vi "Autonomous Independent.vi"   [LabVIEW 2020]
doc: "This VI is called when autonomous begins, and will automatically be terminated when autonomous ends. You can carry out timed or sensor driven robot movement independently without needing to return to the caller."
uses:
  <vilib>/Rock Robotics/Network Tables/NT Read String.vi
  Robot Global Data.vi
panel:
  # "Be sure to right-click and choose Data Operations>>Make Current Value default if you want to save the array values with the VI"
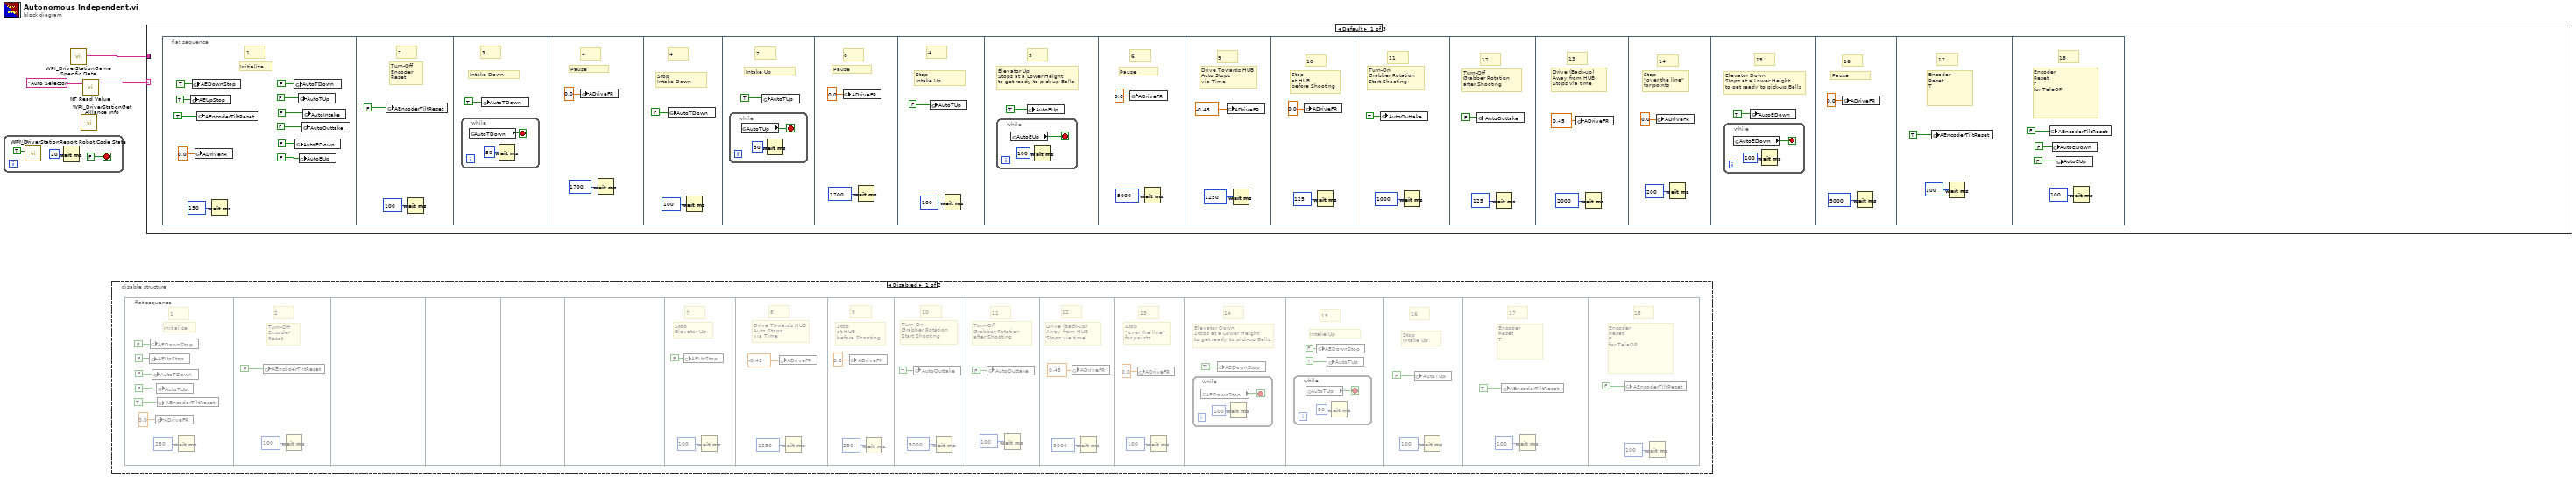
[diagram p0: block diagram]
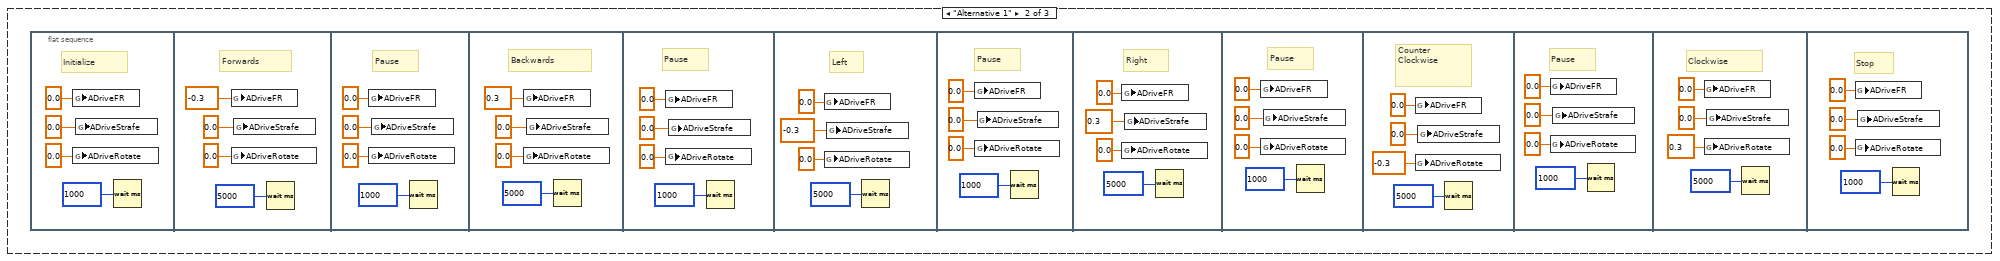
[diagram p3: hidden frame]
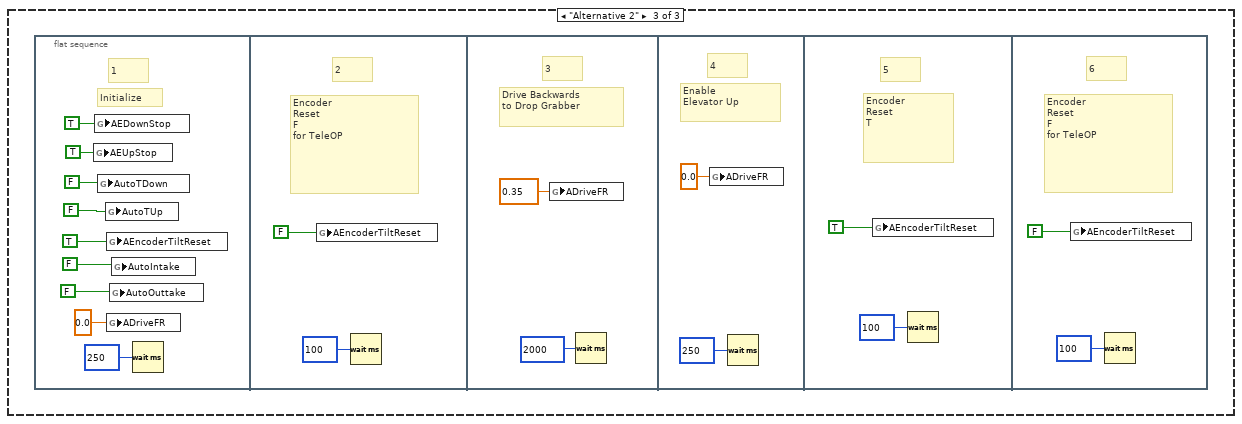
[diagram p4: hidden frame]
diagram:
  n1 = while {
    stop <- FALSE stop-if-true
    n2 = call <vilib>:"WPI_DriverStationReport Robot Code State.vi"("Autonomous"=TRUE) -> ()  [unwired: 10 in, 1 out]
    n3 = Wait (ms)(milliseconds to wait=u32 20) -> ()  [unwired: 1 out]
  }
  n4 = call <vilib>:"WPI_DriverStationGame Specific Data.vi"() -> ("Game Specific Data"=w1:string)  [unwired: 11 in]
  n5 = call <vilib>:"WPI_DriverStationGet Alliance Info.vi"() -> ()  [unwired: 12 out]
  n6 = call-poly <vilib>:"NT Read Value.vi"("Name"="Auto Selector") -> ("String"=w2:string)  [unwired: 9 in, 1 out]
  n7 = disable-structure shown="Disabled" {
    frame Disabled {
      n8 = flat-sequence {
        frame #0 {
          # "1"
          # "Initialize"
          n9 = global write "Robot Global Data.vi" "AEUpStop"(FALSE) -> ()
          n10 = global write "Robot Global Data.vi" "AEDownStop"(FALSE) -> ()
          n11 = global write "Robot Global Data.vi" "AutoTDown"(FALSE) -> ()
          n12 = global write "Robot Global Data.vi" "ADriveFR"(0.0 ("ADriveFR")) -> ()
          n13 = global write "Robot Global Data.vi" "AutoTUp"(FALSE) -> ()
          n14 = global write "Robot Global Data.vi" "AEncoderTiltReset"(TRUE) -> ()
          n15 = Wait (ms)(milliseconds to wait=u32 250) -> ()  [unwired: 1 out]
        }
        frame #1 {
          # "2"
          # "Turn-Off\nEncoder\nReset"
          n16 = global write "Robot Global Data.vi" "AEncoderTiltReset"(FALSE) -> ()
          n17 = Wait (ms)(milliseconds to wait=u32 100) -> ()  [unwired: 1 out]
        }
        frame #2 {
        }
        frame #3 {
        }
        frame #4 {
        }
        frame #5 {
        }
        frame #6 {
          # "7"
          # "Stop\nElevator Up"
          n18 = global write "Robot Global Data.vi" "AEUpStop"(FALSE) -> ()
          n19 = Wait (ms)(milliseconds to wait=u32 100) -> ()  [unwired: 1 out]
        }
        frame #7 {
          # "8"
          # "Drive Towards HUB\nAuto Stops\nvia Time"
          n20 = global write "Robot Global Data.vi" "ADriveFR"(-0.45 ("ADriveFR")) -> ()
          n21 = Wait (ms)(milliseconds to wait=u32 1250) -> ()  [unwired: 1 out]
        }
        frame #8 {
          # "9"
          # "Stop\nat HUB\nbefore Shooting"
          n22 = global write "Robot Global Data.vi" "ADriveFR"(0.0 ("ADriveFR")) -> ()
          n23 = Wait (ms)(milliseconds to wait=u32 250) -> ()  [unwired: 1 out]
        }
        frame #9 {
          # "10"
          # "Turn-On\nGrabber Rotation\nStart Shooting"
          n24 = global write "Robot Global Data.vi" "AutoOuttake"(TRUE ("AutoOuttake")) -> ()
          n25 = Wait (ms)(milliseconds to wait=u32 3000) -> ()  [unwired: 1 out]
        }
        frame #10 {
          # "11"
          # "Turn-Off\nGrabber Rotation\nafter Shooting"
          n26 = global write "Robot Global Data.vi" "AutoOuttake"(FALSE ("AutoOuttake")) -> ()
          n27 = Wait (ms)(milliseconds to wait=u32 100) -> ()  [unwired: 1 out]
        }
        frame #11 {
          # "12"
          # "Drive (Back-up)\nAway from HUB\nStops via time"
          n28 = global write "Robot Global Data.vi" "ADriveFR"(0.45 ("ADriveFR")) -> ()
          n29 = Wait (ms)(milliseconds to wait=u32 3000) -> ()  [unwired: 1 out]
        }
        frame #12 {
          # "13"
          # "Stop\n\"over the line\"\nfor points"
          n30 = global write "Robot Global Data.vi" "ADriveFR"(0.0 ("ADriveFR")) -> ()
          n31 = Wait (ms)(milliseconds to wait=u32 100) -> ()  [unwired: 1 out]
        }
        frame #13 {
          # "14"
          # "Elevator Down\nStops at a Lower Height\nto get ready to pick-up Balls"
          n32 = while {
            stop <- w31 stop-if-true
            n33 = global read "Robot Global Data.vi" "AEDownStop"() -> (w31:bool)
            n34 = Wait (ms)(milliseconds to wait=u32 100) -> ()  [unwired: 1 out]
          }
          n35 = global write "Robot Global Data.vi" "AEDownStop"(TRUE) -> ()
        }
        frame #14 {
          # "Intake Up"
          # "15"
          n36 = while {
            stop <- w35 stop-if-true
            n37 = global read "Robot Global Data.vi" "AutoTUp"() -> (w35:bool)
            n38 = Wait (ms)(milliseconds to wait=u32 50) -> ()  [unwired: 1 out]
          }
          n39 = global write "Robot Global Data.vi" "AEDownStop"(FALSE) -> ()
          n40 = global write "Robot Global Data.vi" "AutoTUp"(TRUE) -> ()
        }
        frame #15 {
          # "Stop\nIntake Up"
          # "16"
          n41 = global write "Robot Global Data.vi" "AutoTUp"(FALSE) -> ()
          n42 = Wait (ms)(milliseconds to wait=u32 100) -> ()  [unwired: 1 out]
        }
        frame #16 {
          # "17"
          # "Encoder\nReset\nT"
          n43 = global write "Robot Global Data.vi" "AEncoderTiltReset"(TRUE) -> ()
          n44 = Wait (ms)(milliseconds to wait=u32 100) -> ()  [unwired: 1 out]
        }
        frame #17 {
          # "18"
          # "Encoder\nReset\nF \nfor TeleOP"
          n45 = global write "Robot Global Data.vi" "AEncoderTiltReset"(FALSE) -> ()
          n46 = Wait (ms)(milliseconds to wait=u32 100) -> ()  [unwired: 1 out]
        }
      }
    }
    frame Enabled {
    }
  }
  n47 = case shown="Default" w2 {
    tunnel: w1 -> [_ _ _]
    frame Default {
      n48 = flat-sequence {
        frame #0 {
          # "1"
          # "Initialize"
          n49 = global write "Robot Global Data.vi" "AEUpStop"(TRUE) -> ()
          n50 = global write "Robot Global Data.vi" "AEDownStop"(TRUE) -> ()
          n51 = global write "Robot Global Data.vi" "ADriveFR"(0.0 ("ADriveFR")) -> ()
          n52 = global write "Robot Global Data.vi" "AEncoderTiltReset"(TRUE) -> ()
          n53 = Wait (ms)(milliseconds to wait=u32 150) -> ()  [unwired: 1 out]
          n54 = global write "Robot Global Data.vi" "AutoTDown"(FALSE) -> ()
          n55 = global write "Robot Global Data.vi" "AutoEDown"(FALSE) -> ()
          n56 = global write "Robot Global Data.vi" "AutoTUp"(FALSE) -> ()
          n57 = global write "Robot Global Data.vi" "AutoEUp"(FALSE) -> ()
          n58 = global write "Robot Global Data.vi" "AutoOuttake"(FALSE) -> ()
          n59 = global write "Robot Global Data.vi" "AutoIntake"(FALSE) -> ()
        }
        frame #1 {
          # "2"
          # "Turn-Off\nEncoder\nReset"
          n60 = global write "Robot Global Data.vi" "AEncoderTiltReset"(FALSE) -> ()
          n61 = Wait (ms)(milliseconds to wait=u32 100) -> ()  [unwired: 1 out]
        }
        frame #2 {
          # "Intake Down"
          # "3"
          n62 = while {
            stop <- w57 stop-if-true
            n63 = global read "Robot Global Data.vi" "AutoTDown"() -> (w57:bool)
            n64 = Wait (ms)(milliseconds to wait=u32 50) -> ()  [unwired: 1 out]
          }
          n65 = global write "Robot Global Data.vi" "AutoTDown"(TRUE) -> ()
        }
        frame #3 {
          # "4"
          # "Pause"
          n66 = global write "Robot Global Data.vi" "ADriveFR"(0.0 ("ADriveFR")) -> ()
          n67 = Wait (ms)(milliseconds to wait=u32 1700) -> ()  [unwired: 1 out]
        }
        frame #4 {
          # "Stop \nIntake Down"
          # "4"
          n68 = global write "Robot Global Data.vi" "AutoTDown"(FALSE) -> ()
          n69 = Wait (ms)(milliseconds to wait=u32 100) -> ()  [unwired: 1 out]
        }
        frame #5 {
          # "Intake Up"
          # "7"
          n70 = while {
            stop <- w64 stop-if-true
            n71 = global read "Robot Global Data.vi" "AutoTUp"() -> (w64:bool)
            n72 = Wait (ms)(milliseconds to wait=u32 50) -> ()  [unwired: 1 out]
          }
          n73 = global write "Robot Global Data.vi" "AutoTUp"(TRUE) -> ()
        }
        frame #6 {
          # "8"
          # "Pause"
          n74 = global write "Robot Global Data.vi" "ADriveFR"(0.0 ("ADriveFR")) -> ()
          n75 = Wait (ms)(milliseconds to wait=u32 1700) -> ()  [unwired: 1 out]
        }
        frame #7 {
          # "Stop \nIntake Up"
          # "4"
          n76 = global write "Robot Global Data.vi" "AutoTUp"(FALSE) -> ()
          n77 = Wait (ms)(milliseconds to wait=u32 100) -> ()  [unwired: 1 out]
        }
        frame #8 {
          # "5"
          # "Elevator Up\nStops at a Lower Height\nto get ready to pick-up Balls"
          n78 = while {
            stop <- w71 stop-if-true
            n79 = global read "Robot Global Data.vi" "AutoEUp"() -> (w71:bool)
            n80 = Wait (ms)(milliseconds to wait=u32 100) -> ()  [unwired: 1 out]
          }
          n81 = global write "Robot Global Data.vi" "AutoEUp"(TRUE) -> ()
        }
        frame #9 {
          # "6"
          # "Pause"
          n82 = global write "Robot Global Data.vi" "ADriveFR"(0.0 ("ADriveFR")) -> ()
          n83 = Wait (ms)(milliseconds to wait=u32 5000) -> ()  [unwired: 1 out]
        }
        frame #10 {
          # "9"
          # "Drive Towards HUB\nAuto Stops\nvia Time"
          n84 = global write "Robot Global Data.vi" "ADriveFR"(-0.45 ("ADriveFR")) -> ()
          n85 = Wait (ms)(milliseconds to wait=u32 1250) -> ()  [unwired: 1 out]
        }
        frame #11 {
          # "10"
          # "Stop\nat HUB\nbefore Shooting"
          n86 = global write "Robot Global Data.vi" "ADriveFR"(0.0 ("ADriveFR")) -> ()
          n87 = Wait (ms)(milliseconds to wait=u32 125) -> ()  [unwired: 1 out]
        }
        frame #12 {
          # "11"
          # "Turn-On\nGrabber Rotation\nStart Shooting"
          n88 = global write "Robot Global Data.vi" "AutoOuttake"(TRUE ("AutoOuttake")) -> ()
          n89 = Wait (ms)(milliseconds to wait=u32 1000) -> ()  [unwired: 1 out]
        }
        frame #13 {
          # "12"
          # "Turn-Off\nGrabber Rotation\nafter Shooting"
          n90 = global write "Robot Global Data.vi" "AutoOuttake"(FALSE ("AutoOuttake")) -> ()
          n91 = Wait (ms)(milliseconds to wait=u32 125) -> ()  [unwired: 1 out]
        }
        frame #14 {
          # "13"
          # "Drive (Back-up)\nAway from HUB\nStops via time"
          n92 = global write "Robot Global Data.vi" "ADriveFR"(0.45 ("ADriveFR")) -> ()
          n93 = Wait (ms)(milliseconds to wait=u32 2000) -> ()  [unwired: 1 out]
        }
        frame #15 {
          # "14"
          # "Stop\n\"over the line\"\nfor points"
          n94 = global write "Robot Global Data.vi" "ADriveFR"(0.0 ("ADriveFR")) -> ()
          n95 = Wait (ms)(milliseconds to wait=u32 200) -> ()  [unwired: 1 out]
        }
        frame #16 {
          # "15"
          # "Elevator Down\nStops at a Lower Height\nto get ready to pick-up Balls"
          n96 = while {
            stop <- w88 stop-if-true
            n97 = global read "Robot Global Data.vi" "AutoEDown"() -> (w88:bool)
            n98 = Wait (ms)(milliseconds to wait=u32 100) -> ()  [unwired: 1 out]
          }
          n99 = global write "Robot Global Data.vi" "AutoEDown"(TRUE) -> ()
        }
        frame #17 {
          # "16"
          # "Pause"
          n100 = global write "Robot Global Data.vi" "ADriveFR"(0.0 ("ADriveFR")) -> ()
          n101 = Wait (ms)(milliseconds to wait=u32 5000) -> ()  [unwired: 1 out]
        }
        frame #18 {
          # "17"
          # "Encoder\nReset\nT"
          n102 = global write "Robot Global Data.vi" "AEncoderTiltReset"(TRUE) -> ()
          n103 = Wait (ms)(milliseconds to wait=u32 100) -> ()  [unwired: 1 out]
        }
        frame #19 {
          # "18"
          # "Encoder\nReset\nF \nfor TeleOP"
          n104 = global write "Robot Global Data.vi" "AEncoderTiltReset"(FALSE) -> ()
          n105 = global write "Robot Global Data.vi" "AutoEDown"(FALSE) -> ()
          n106 = global write "Robot Global Data.vi" "AutoEUp"(FALSE) -> ()
          n107 = Wait (ms)(milliseconds to wait=u32 100) -> ()  [unwired: 1 out]
        }
      }
    }
    frame "Alternative 1" {
      n108 = flat-sequence {
        frame #0 {
          # "Initialize"
          n109 = global write "Robot Global Data.vi" "ADriveFR"(0.0 ("ADriveFR")) -> ()
          n110 = global write "Robot Global Data.vi" "ADriveRotate"(0.0 ("ADriveRotate")) -> ()
          n111 = global write "Robot Global Data.vi" "ADriveStrafe"(0.0 ("ADriveLStrafe")) -> ()
          n112 = Wait (ms)(milliseconds to wait=u32 1000) -> ()  [unwired: 1 out]
        }
        frame #1 {
          # "Forwards"
          n113 = global write "Robot Global Data.vi" "ADriveFR"(-0.3 ("ADriveFR")) -> ()
          n114 = global write "Robot Global Data.vi" "ADriveRotate"(0.0 ("ADriveRotate")) -> ()
          n115 = global write "Robot Global Data.vi" "ADriveStrafe"(0.0 ("ADriveLStrafe")) -> ()
          n116 = Wait (ms)(milliseconds to wait=u32 5000) -> ()  [unwired: 1 out]
        }
        frame #2 {
          # "Pause"
          n117 = global write "Robot Global Data.vi" "ADriveFR"(0.0 ("ADriveFR")) -> ()
          n118 = global write "Robot Global Data.vi" "ADriveRotate"(0.0 ("ADriveRotate")) -> ()
          n119 = global write "Robot Global Data.vi" "ADriveStrafe"(0.0 ("ADriveLStrafe")) -> ()
          n120 = Wait (ms)(milliseconds to wait=u32 1000) -> ()  [unwired: 1 out]
        }
        frame #3 {
          # "Backwards"
          n121 = global write "Robot Global Data.vi" "ADriveFR"(0.3 ("ADriveFR")) -> ()
          n122 = global write "Robot Global Data.vi" "ADriveRotate"(0.0 ("ADriveRotate")) -> ()
          n123 = global write "Robot Global Data.vi" "ADriveStrafe"(0.0 ("ADriveLStrafe")) -> ()
          n124 = Wait (ms)(milliseconds to wait=u32 5000) -> ()  [unwired: 1 out]
        }
        frame #4 {
          # "Pause"
          n125 = global write "Robot Global Data.vi" "ADriveFR"(0.0 ("ADriveFR")) -> ()
          n126 = global write "Robot Global Data.vi" "ADriveRotate"(0.0 ("ADriveRotate")) -> ()
          n127 = global write "Robot Global Data.vi" "ADriveStrafe"(0.0 ("ADriveLStrafe")) -> ()
          n128 = Wait (ms)(milliseconds to wait=u32 1000) -> ()  [unwired: 1 out]
        }
        frame #5 {
          # "Left"
          n129 = global write "Robot Global Data.vi" "ADriveFR"(0.0 ("ADriveFR")) -> ()
          n130 = global write "Robot Global Data.vi" "ADriveRotate"(0.0 ("ADriveRotate")) -> ()
          n131 = global write "Robot Global Data.vi" "ADriveStrafe"(-0.3 ("ADriveLStrafe")) -> ()
          n132 = Wait (ms)(milliseconds to wait=u32 5000) -> ()  [unwired: 1 out]
        }
        frame #6 {
          # "Pause"
          n133 = global write "Robot Global Data.vi" "ADriveFR"(0.0 ("ADriveFR")) -> ()
          n134 = global write "Robot Global Data.vi" "ADriveRotate"(0.0 ("ADriveRotate")) -> ()
          n135 = global write "Robot Global Data.vi" "ADriveStrafe"(0.0 ("ADriveLStrafe")) -> ()
          n136 = Wait (ms)(milliseconds to wait=u32 1000) -> ()  [unwired: 1 out]
        }
        frame #7 {
          # "Right"
          n137 = global write "Robot Global Data.vi" "ADriveFR"(0.0 ("ADriveFR")) -> ()
          n138 = global write "Robot Global Data.vi" "ADriveRotate"(0.0 ("ADriveRotate")) -> ()
          n139 = global write "Robot Global Data.vi" "ADriveStrafe"(0.3 ("ADriveLStrafe")) -> ()
          n140 = Wait (ms)(milliseconds to wait=u32 5000) -> ()  [unwired: 1 out]
        }
        frame #8 {
          # "Pause"
          n141 = global write "Robot Global Data.vi" "ADriveFR"(0.0 ("ADriveFR")) -> ()
          n142 = global write "Robot Global Data.vi" "ADriveRotate"(0.0 ("ADriveRotate")) -> ()
          n143 = global write "Robot Global Data.vi" "ADriveStrafe"(0.0 ("ADriveLStrafe")) -> ()
          n144 = Wait (ms)(milliseconds to wait=u32 1000) -> ()  [unwired: 1 out]
        }
        frame #9 {
          # "Counter\nClockwise"
          n145 = global write "Robot Global Data.vi" "ADriveFR"(0.0 ("ADriveFR")) -> ()
          n146 = global write "Robot Global Data.vi" "ADriveRotate"(-0.3 ("ADriveRotate")) -> ()
          n147 = global write "Robot Global Data.vi" "ADriveStrafe"(0.0 ("ADriveLStrafe")) -> ()
          n148 = Wait (ms)(milliseconds to wait=u32 5000) -> ()  [unwired: 1 out]
        }
        frame #10 {
          # "Pause"
          n149 = global write "Robot Global Data.vi" "ADriveFR"(0.0 ("ADriveFR")) -> ()
          n150 = global write "Robot Global Data.vi" "ADriveRotate"(0.0 ("ADriveRotate")) -> ()
          n151 = global write "Robot Global Data.vi" "ADriveStrafe"(0.0 ("ADriveLStrafe")) -> ()
          n152 = Wait (ms)(milliseconds to wait=u32 1000) -> ()  [unwired: 1 out]
        }
        frame #11 {
          # "Clockwise"
          n153 = global write "Robot Global Data.vi" "ADriveFR"(0.0 ("ADriveFR")) -> ()
          n154 = global write "Robot Global Data.vi" "ADriveRotate"(0.3 ("ADriveRotate")) -> ()
          n155 = global write "Robot Global Data.vi" "ADriveStrafe"(0.0 ("ADriveLStrafe")) -> ()
          n156 = Wait (ms)(milliseconds to wait=u32 5000) -> ()  [unwired: 1 out]
        }
        frame #12 {
          # "Stop"
          n157 = global write "Robot Global Data.vi" "ADriveFR"(0.0 ("ADriveFR")) -> ()
          n158 = global write "Robot Global Data.vi" "ADriveRotate"(0.0 ("ADriveRotate")) -> ()
          n159 = global write "Robot Global Data.vi" "ADriveStrafe"(0.0 ("ADriveLStrafe")) -> ()
          n160 = Wait (ms)(milliseconds to wait=u32 1000) -> ()  [unwired: 1 out]
        }
      }
    }
    frame "Alternative 2" {
      n161 = flat-sequence {
        frame #0 {
          # "1"
          # "Initialize"
          n162 = global write "Robot Global Data.vi" "AEUpStop"(TRUE) -> ()
          n163 = global write "Robot Global Data.vi" "AEDownStop"(TRUE) -> ()
          n164 = global write "Robot Global Data.vi" "AutoTDown"(FALSE) -> ()
          n165 = global write "Robot Global Data.vi" "AutoTUp"(FALSE) -> ()
          n166 = global write "Robot Global Data.vi" "AEncoderTiltReset"(TRUE) -> ()
          n167 = global write "Robot Global Data.vi" "ADriveFR"(0.0 ("ADriveFR")) -> ()
          n168 = global write "Robot Global Data.vi" "AutoOuttake"(FALSE) -> ()
          n169 = global write "Robot Global Data.vi" "AutoIntake"(FALSE) -> ()
          n170 = Wait (ms)(milliseconds to wait=u32 250) -> ()  [unwired: 1 out]
        }
        frame #1 {
          # "2"
          # "Encoder\nReset\nF \nfor TeleOP"
          n171 = global write "Robot Global Data.vi" "AEncoderTiltReset"(FALSE) -> ()
          n172 = Wait (ms)(milliseconds to wait=u32 100) -> ()  [unwired: 1 out]
        }
        frame #2 {
          # "3"
          # "Drive Backwards\nto Drop Grabber"
          n173 = global write "Robot Global Data.vi" "ADriveFR"(0.35 ("ADriveFR")) -> ()
          n174 = Wait (ms)(milliseconds to wait=u32 2000) -> ()  [unwired: 1 out]
        }
        frame #3 {
          # "4"
          # "Enable\nElevator Up"
          n175 = global write "Robot Global Data.vi" "ADriveFR"(0.0 ("ADriveFR")) -> ()
          n176 = Wait (ms)(milliseconds to wait=u32 250) -> ()  [unwired: 1 out]
        }
        frame #4 {
          # "5"
          # "Encoder\nReset\nT"
          n177 = global write "Robot Global Data.vi" "AEncoderTiltReset"(TRUE) -> ()
          n178 = Wait (ms)(milliseconds to wait=u32 100) -> ()  [unwired: 1 out]
        }
        frame #5 {
          # "6"
          # "Encoder\nReset\nF \nfor TeleOP"
          n179 = global write "Robot Global Data.vi" "AEncoderTiltReset"(FALSE) -> ()
          n180 = Wait (ms)(milliseconds to wait=u32 100) -> ()  [unwired: 1 out]
        }
      }
    }
  }
